vi "Reconnect.vi"(8 "error in (no error)":errorcluster, 11 "BaseDriver in":refnum<class "BaseDriver.lvclass">) -> (0 "error out":errorcluster, 3 "BaseDriver out":refnum<class "BaseDriver.lvclass">)   [LabVIEW 2025, in "BaseDriver.lvclass"]
doc: "Called when the driver has lost connection to the remote destination. Will try to reconnect and emits a reconnected response if sucessful"
uses:
  BaseDriver.lvclass
  BaseDriver.lvclass/BaseDriver.ctl
  response.ctl
  driver_status.ctl
  Reader/BaseReader/BaseReader.lvclass
  Responder/BaseResponder/BaseResponder.lvclass
  <userlib>/_OpenG.lib/time/time.llb/openg_time.lvlib
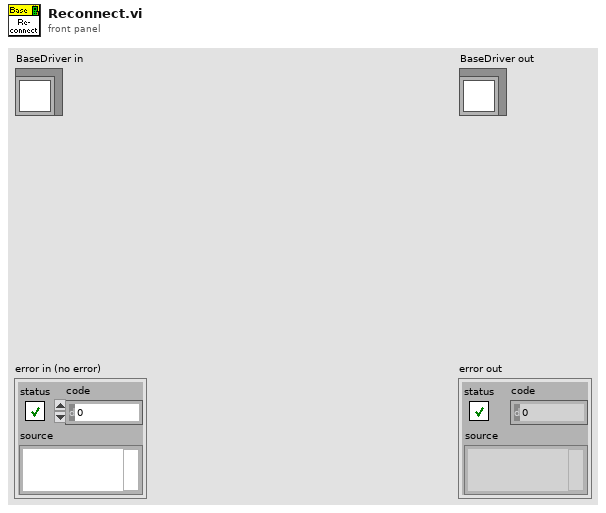
[diagram p1: front panel]
types:
  T1 = typedef "response.ctl" = cluster{"driver status":T2, "Sender":string, "Type":i32, "Variant":variant}
  T2 = typedef "driver_status.ctl" = enum16{"Normal", "Startup", "Connection lost", "Reconnected", "Timeout", "Idle", "Busy"}
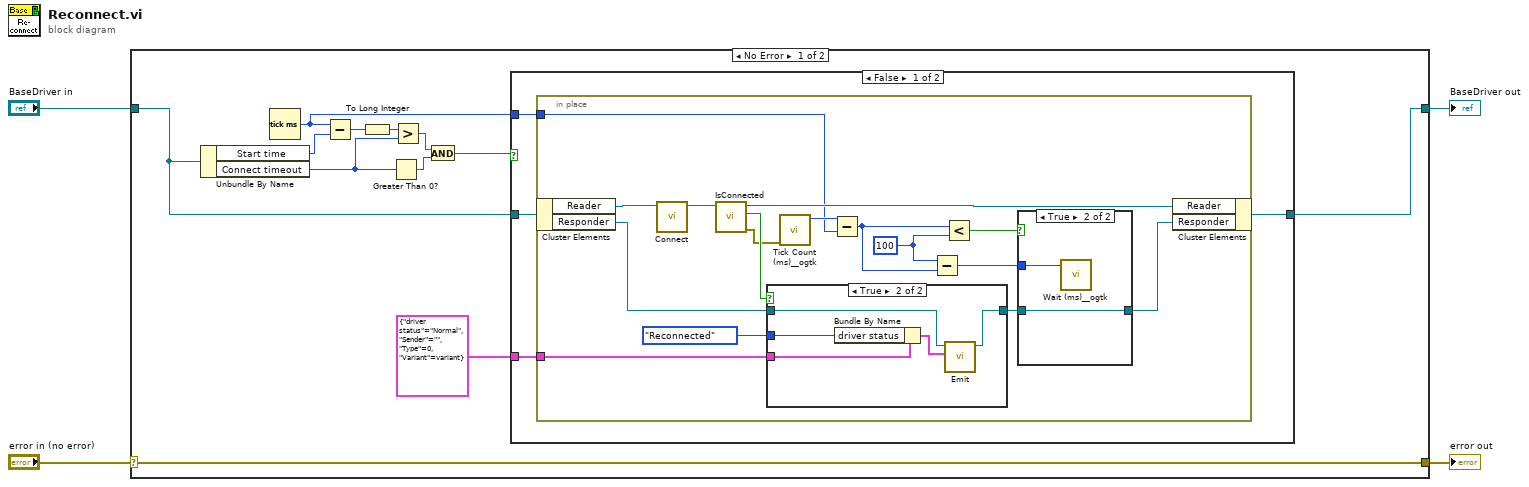
[diagram p0: block diagram]
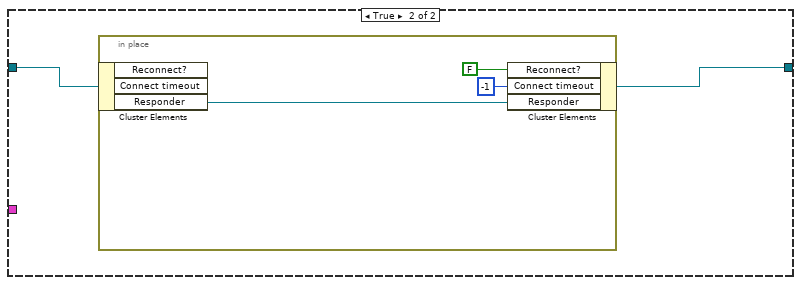
[diagram p4: hidden frame]
diagram:
  n1 = case shown="No Error" "error in (no error)" {
    selector: "error in (no error)" -> [w16 w52]
    tunnel: [w16 w52] -> w3
    tunnel: [w15 w51] -> w1
    tunnel: "BaseDriver in" -> [w7 w51]
    frame No Error {
      n2 = Unbundle By Name(w7) -> ("Start time"=w13:u32, "Connect timeout"=w12:i32)
      n3 = Tick Count (ms)() -> (millisecond timer value=w6:u32)
      n4 = Subtract(x=w6, y=w13) -> (x-y=w14:u32)
      n5 = To Long Integer(number=w14) -> (32bit integer=w9:i32)
      n6 = Greater Than 0?(x=w12) -> (x > 0?=w10:bool)
      n7 = Greater?(x=w9, y=w12) -> (0:w11:bool)
      n8 = And(x=w11, y=w10) -> (x .and. y?=w8:bool)
      n9 = case shown="False" w8 {
        tunnel: [w20 w46] -> w15
        tunnel: w7 -> [w19 w47]
        tunnel: w6 -> [w18 _]
        tunnel: T1 {"driver status"=enum."Normal", "Sender"="", "Type"=0, "Variant"=variant} ("response") -> [w17 _]
        frame False {
          n10 = in-place "In Place Element Structure" {
            in-place-border: w18 -> [w23]
            in-place-border: w17 -> [w22]
            w25 = u32 100 ("y")
            n11 = in-place-cluster #1(w19) -> ("Reader"=w36:refnum<class "BaseReader.lvclass">, "Responder"=w32:refnum<class "BaseResponder.lvclass">)
            n12 = call-dynamic "Connect.vi"("BaseReader in"=w36) -> ("BaseReader out"=w34:refnum<class "BaseReader.lvclass">)  [unwired: 9 in, 1 out]
            n13 = call-dynamic "IsConnected.vi"("BaseReader in"=w34) -> ("error out"=w31:errorcluster, "connected?"=w35:bool, "BaseReader out"=w33:refnum<class "BaseReader.lvclass">)  [unwired: 8 in]
            n14 = case shown="True" w35 {
              tunnel: w32 -> [w40 w45]
              tunnel: [w40 w44] -> w28
              tunnel: w22 -> [_ w43]
              tunnel: driver_status."Reconnected" ("driver status") -> [_ w41]
              frame False {
              }
              frame True {
                n15 = Bundle By Name(cluster=w43, "driver status"=w41) -> (w42:T1)
                n16 = call-dynamic "Emit.vi"("response"=w42, "BaseResponder in"=w45) -> ("BaseResponder out"=w44:refnum<class "BaseResponder.lvclass">)  [unwired: 8 in, 1 out]
              }
            }
            n17 = call <userlib>:"Tick Count (ms)__ogtk.vi"("error in (no error)"=w31) -> ("millisecond timer value"=w30:u32)  [unwired: 9 in, 1 out]
            n18 = Subtract(x=w30, y=w23) -> (x-y=w24:u32)
            n19 = Subtract(x=w25, y=w24) -> (x-y=w26:u32)
            n20 = Less?(x=w24, y=w25) -> (x < y?=w27:bool)
            n21 = case shown="True" w27 {
              tunnel: w26 -> [_ w38]
              tunnel: [w37 w39] -> w29
              tunnel: w28 -> [w37 w39]
              frame False {
              }
              frame True {
                n22 = call <userlib>:"Wait (ms)__ogtk.vi"("milliseconds to wait"=w38) -> ()  [unwired: 9 in, 2 out]
              }
            }
            n23 = in-place-cluster #1("Reader"=w33, "Responder"=w29) -> (w20:refnum<class "BaseDriver.lvclass">)
          }
        }
        frame True {
          n24 = in-place "In Place Element Structure" {
            n25 = in-place-cluster #2(w47) -> ("Responder"=w48:refnum<class "BaseResponder.lvclass">)  [unwired: 2 out]
            n26 = in-place-cluster #2("Reconnect?"=FALSE, "Connect timeout"=-1, "Responder"=w48) -> (w46:refnum<class "BaseDriver.lvclass">)
          }
        }
      }
    }
    frame Error {
    }
  }
  "error out" <- w3
  "BaseDriver out" <- w1
